vi "Read dblEventSignalArray.vi"(8 "error in (no error)":errorcluster, 11 "EventPluginBaseClass in":refnum<class "BaseWfrmPlugin.lvclass">) -> (0 "error out":errorcluster, 2 "dblEventSignalArray":T1, 3 "EventPluginBaseClass out":refnum<class "BaseWfrmPlugin.lvclass">)   [LabVIEW 2014, in "WfrmPlugins.lvlib" / "BaseWfrmPlugin.lvclass"]
uses:
  BaseWfrmPlugin.lvclass
  TypeDefs/dblEvtSignalArray.ctl
  BaseWfrmPlugin.lvclass/BaseWfrmPlugin.ctl
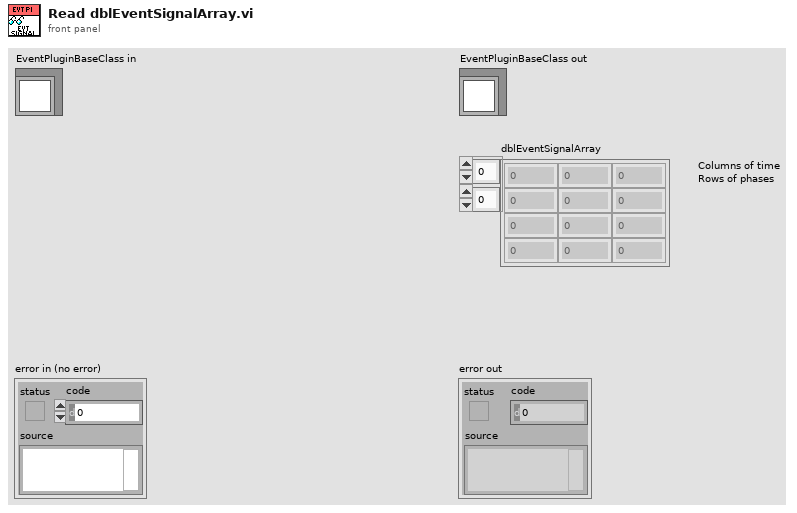
[diagram p1: front panel]
types:
  T1 = typedef "WfrmPlugins.lvlib/BaseWfrmPlugin.lvclass/dblEvtSignalArray.ctl" = dbl[][]
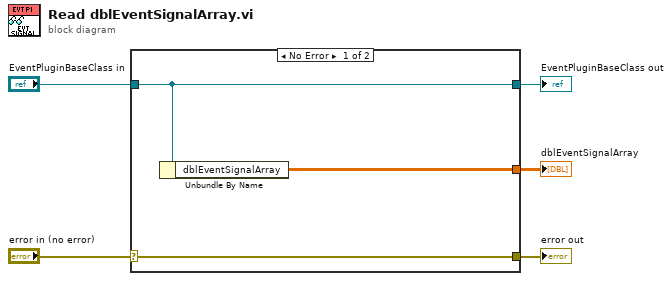
[diagram p0: block diagram]
diagram:
  n1 = case shown="No Error" "error in (no error)" {
    selector: "error in (no error)" -> [w8 w9]
    tunnel: [w8 w9] -> w4
    tunnel: [w7 w10] -> w2
    tunnel: "EventPluginBaseClass in" -> [w7 w10]
    tunnel: [w6 _] -> w1
    frame No Error {
      n2 = Unbundle By Name(w7) -> ("dblEventSignalArray"=w6:T1)
    }
    frame Error {
    }
  }
  "error out" <- w4
  "EventPluginBaseClass out" <- w2
  "dblEventSignalArray" <- w1
